vi "Test Generate Mock Class Creates Constructor.vi"(8 "error in (no error)":errorcluster, 11 "Test Case In":refnum<class "Mock Class Generator Test.lvclass">) -> (0 "error out":errorcluster, 3 "Test Case Out":refnum<class "Mock Class Generator Test.lvclass">)   [LabVIEW 2020, in "Mock Class Generator Test.lvclass"]
uses:
  Mock Class Generator Test.lvclass
  C:/Program Files (x86)/National Instruments/LabVIEW 2020/vi.lib/Astemes/LUnit/Test Case.lvclass
  <vilib>/Astemes/LUnit/Test Case.lvclass/Test Case.ctl
  <vilib>/Astemes/LUnit/Append Fail Result.vi
  <vilib>/Astemes/LUnit/Append Pass Result.vi
  source/Scripting/Mock Class Generator/Mock Class Generator.lvclass
  <vilib>/Astemes/LUnit/Test Case.lvclass
panel:
  out "file or folder exists?":bool
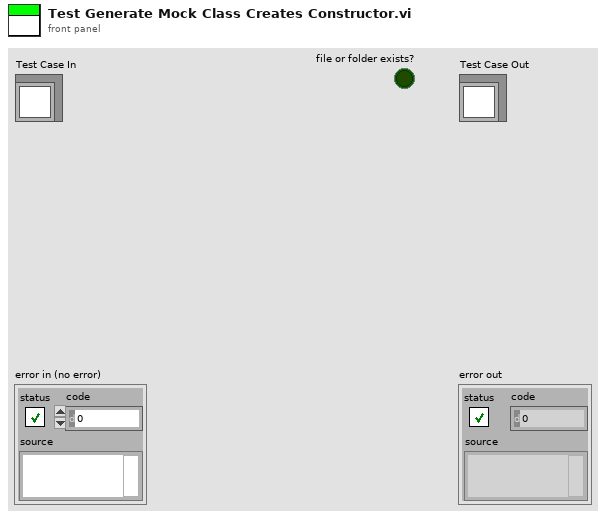
[diagram p1: front panel]
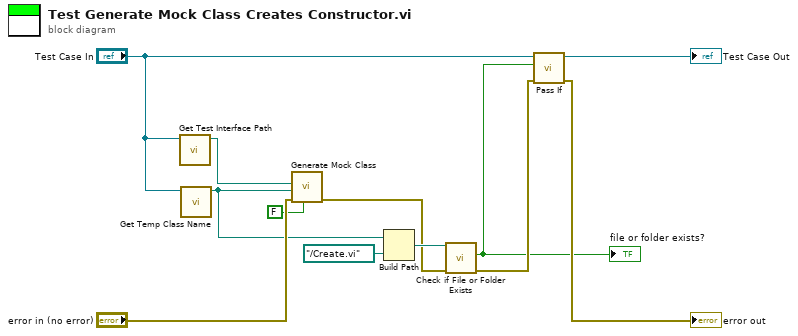
[diagram p0: block diagram]
diagram:
  n1 = call "Get Test Interface Path.vi"("Mock Class Generator Test in"="Test Case In") -> ("Test Class Path"=w10:path)  [unwired: 10 in]
  n2 = call "Get Temp Class Name.vi"("Mock Class Generator Test in"="Test Case In") -> ("Test Class Path"=w6:path)  [unwired: 10 in]
  n3 = call "Generate Mock Class.vi"("Add to lvproj?"=FALSE, "error in (no error)"="error in (no error)", "Destination Class Path"=w6, "Source Class Path"=w10) -> ("error out"=w3:errorcluster)  [unwired: 7 in]
  n4 = Build Path(base path=w6, name or relative path=path "../Create.vi") -> (appended path=w4:path)
  n5 = call <vilib>:"Check if File or Folder Exists.vi"("error in (no error)"=w3, "path"=w4) -> ("error out"=w2:errorcluster, "file or folder exists?"=w1:bool)  [unwired: 7 in, 1 out]
  "file or folder exists?" <- w1
  n6 = call <vilib>:"Pass If.vi"("error in (no error)"=w2, "Pass?"=w1, "LUnit Test Case In"="Test Case In") -> ("error out"=→"error out":errorcluster, "LUnit Test Case Out"=→"Test Case Out":refnum<class "Mock Class Generator Test.lvclass">)  [unwired: 7 in]
